vi "Wait for Operation Complete.vi"(8 "error in (no error)":errorcluster, 9 "Maximum Time (10000 ms)":i32=10000, 10 "Channel (0: Channel 1)":i32(ring) items=["Channel 1", "Channel 2"], 11 "VISA resource name":refnum<visa-resource-name>) -> (0 "error out":errorcluster, 3 "VISA resource name out":refnum<visa-resource-name>)   [LabVIEW 2020, in "Agilent B2900 Series.lvlib"]
doc: "Waits for all the operation to finish.\n\n<B>Note:</B> \n(1) Use this VI only with other low-level VIs. This VI does not check the instrument status."
uses:
  Agilent B2900 Series.lvlib
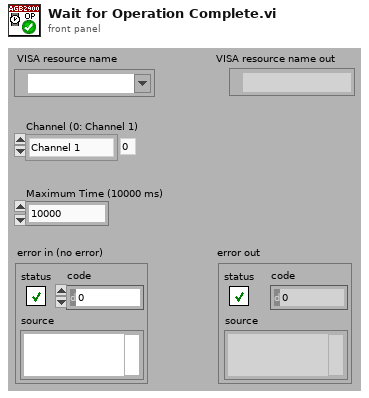
[diagram p1: front panel]
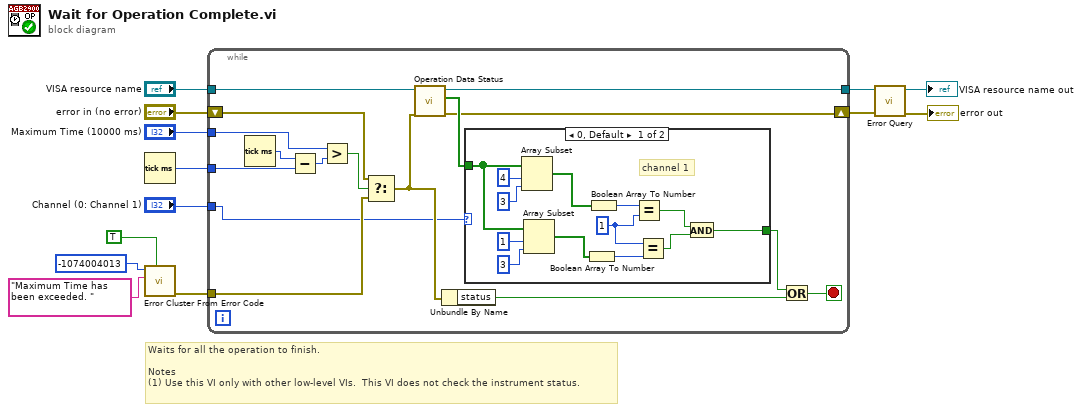
[diagram p0: block diagram]
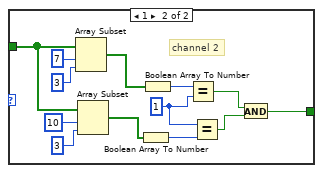
[diagram p2: hidden frame]
diagram:
  # "Waits for all the operation to finish.\n\nNotes\n(1) Use this VI only with other low-level VIs.  This VI does not check the instrument status."
  n1 = Tick Count (ms)() -> (millisecond timer value=w9:u32)
  n2 = call <vilib>:"Error Cluster From Error Code.vi"("show call chain? (False)"=TRUE, "error message (\"\")"="Maximum Time has been exceeded. " ("error message (\"\")"), "error code (0)"=-1074004013) -> ("error out"=w11:errorcluster)  [unwired: 6 in]
  n3 = while {
    tunnel: w11 -> [w25]
    tunnel: w9 -> [w28]
    tunnel: "Maximum Time (10000 ms)" -> [w27]
    shift-right: [w17] -> w2
    shift-left: "error in (no error)" -> [w23]
    tunnel: [w18] -> w3
    tunnel: "VISA resource name" -> [w19]
    tunnel: "Channel (0: Channel 1)" -> [w14]
    stop <- w24 stop-if-true
    n4 = Tick Count (ms)() -> (millisecond timer value=w29:u32)
    n5 = Subtract(x=w29, y=w28) -> (x-y=w26:u32)
    n6 = Greater?(x=w27, y=w26) -> (0:w22:bool)
    n7 = Select(t=w23, s=w22, f=w25) -> (s? t:f=w16:errorcluster)
    n8 = call "Operation Data Status.vi"("error in (no error)"=w16, "VISA resource name"=w19) -> ("error out"=w17:errorcluster, "Operation Register Status"=w20:bool[], "VISA resource name out"=w18:refnum<visa-resource-name>)  [unwired: 7 in]
    n9 = Unbundle By Name(w16) -> ("status"=w21:bool)
    n10 = case shown="0, Default" w14 {
      tunnel: w20 -> [w40 w43]
      tunnel: [w30 w44] -> w15
      frame 0, Default {
        w33 = u32 1 ("y")
        # "channel 1"
        n11 = Array Subset(array=w40, index=4, length=3) -> (w36:bool[])
        n12 = Array Subset(array=w40, index=1, length=3) -> (w34:bool[])
        n13 = Boolean Array To Number(Boolean array=w34) -> (number=w35:u32)
        n14 = Boolean Array To Number(Boolean array=w36) -> (number=w37:u32)
        n15 = Equal?(x=w37, y=w33) -> (x = y?=w32:bool)
        n16 = Equal?(x=w33, y=w35) -> (x = y?=w31:bool)
        n17 = And(x=w32, y=w31) -> (x .and. y?=w30:bool)
      }
      frame 1 {
        w47 = u32 1 ("y")
        # "channel 2"
        n18 = Array Subset(array=w43, index=7, length=3) -> (w50:bool[])
        n19 = Array Subset(array=w43, index=10, length=3) -> (w48:bool[])
        n20 = Boolean Array To Number(Boolean array=w48) -> (number=w49:u32)
        n21 = Boolean Array To Number(Boolean array=w50) -> (number=w51:u32)
        n22 = Equal?(x=w51, y=w47) -> (x = y?=w46:bool)
        n23 = Equal?(x=w47, y=w49) -> (x = y?=w45:bool)
        n24 = And(x=w46, y=w45) -> (x .and. y?=w44:bool)
      }
    }
    n25 = Or(x=w15, y=w21) -> (x .or. y?=w24:bool)
  }
  n26 = call "Error Query.vi"("error in (no error)"=w2, "VISA resource name"=w3) -> ("error out"=→"error out":errorcluster, "VISA resource name out"=→"VISA resource name out":refnum<visa-resource-name>)  [unwired: 6 in, 2 out]
